vi "GV_Joystick1.vi"(8 "error in (no error)":errorcluster, 10 "device index":i32, 11 "Mode":enum16{"Init", "Destroy", "Read", "Change ID"}(ring)) -> (0 "error out":errorcluster, 1 "Connected?":bool, 2 "device":refnum<k1>, 3 "device ID":i32)   [LabVIEW 2012]
uses:
  <vilib>/Utility/inputDevices.llb/closeJoystick.vi
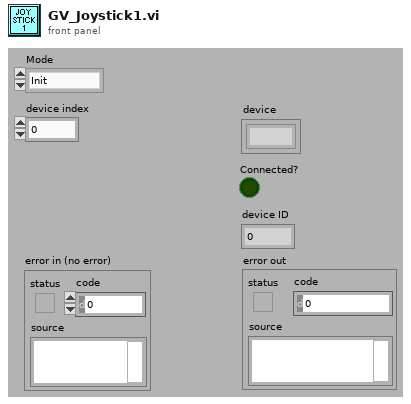
[diagram p1: front panel]
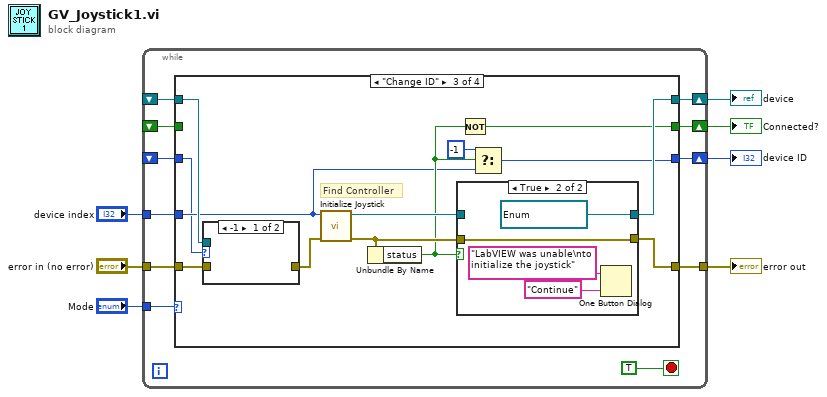
[diagram p0: block diagram]
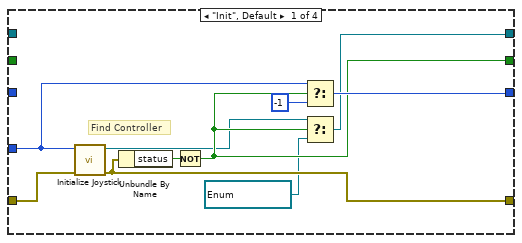
[diagram p2: hidden frame]
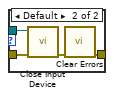
[diagram p4: hidden frame]
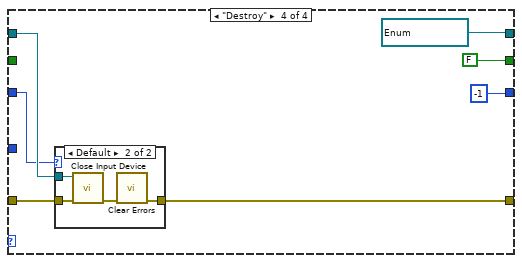
[diagram p6: hidden frame]
diagram:
  n1 = while {
    shift-right: [w18] -> w4
    shift-left: _ -> [w16]
    shift-right: [w17] -> w3
    shift-left: _ -> [w15]
    shift-right: [w13] -> w2
    shift-left: _ -> [w12]
    tunnel: "device index" -> [w11]
    tunnel: "Mode" -> [w10]
    tunnel: "error in (no error)" -> [w9]
    tunnel: [w8] -> w1
    stop <- TRUE stop-if-true
    n2 = case shown="\"Change ID\"" w10 {
      tunnel: [w20 w32 w43 w60] -> w18
      tunnel: [w22 w31 w41 FALSE] -> w17
      tunnel: w16 -> [_ w32 w40 w62]
      tunnel: w15 -> [_ w31 _ _]
      tunnel: w11 -> [w25 _ w34 _]
      tunnel: w9 -> [w27 w30 w39 w61]
      tunnel: [w28 w30 w42 w58] -> w8
      tunnel: [w23 w29 w36 -1 ("f")] -> w13
      tunnel: w12 -> [_ w29 w33 w56]
      frame "Init", Default {
        w19 = refnum<k1> refnum items=["JOYSTICK"] ("device ID")
        # "Find Controller"
        n3 = call <vilib>:"Initialize Joystick.vi"("error in (no error)"=w27, "device index"=w25) -> ("error out"=w28:errorcluster, "device ID"=w21:refnum<k1>)  [unwired: 8 in]
        n4 = Unbundle By Name(w28) -> ("status"=w26:bool)
        n5 = Not(x=w26) -> (.not. x?=w22:bool)
        n6 = Select(t=w25, s=w22, f=-1) -> (s? t:f=w23:i32)
        n7 = Select(t=w21, s=w22, f=w19) -> (s? t:f=w20:refnum<k1>)
      }
      frame "Read" {
      }
      frame "Change ID" {
        # "Find Controller"
        n8 = case shown="-1" w33 {
          tunnel: w40 -> [_ w49]
          tunnel: w39 -> [_ w48]
          tunnel: [_ w46] -> w38
          frame -1 {
          }
          frame Default {
            n9 = call-poly <vilib>:"Close Input Device.vi"("error in (no error)"=w48, "device ID"=w49) -> ("error out"=w47:errorcluster)  [unwired: 8 in]
            n10 = call <vilib>:"Clear Errors.vi"("error in (no error)"=w47) -> ("error out"=w46:errorcluster)  [unwired: 6 in]
          }
        }
        n11 = call <vilib>:"Initialize Joystick.vi"("error in (no error)"=w38, "device index"=w34) -> ("error out"=w45:errorcluster, "device ID"=w44:refnum<k1>)  [unwired: 8 in]
        n12 = Unbundle By Name(w45) -> ("status"=w37:bool)
        n13 = case shown="True" w37 {
          tunnel: w45 -> [w51 w53]
          tunnel: [w51 w53] -> w42
          tunnel: w44 -> [w50 _]
          tunnel: [w50 w52] -> w43
          frame False {
          }
          frame True {
            w52 = refnum<k1> refnum items=["JOYSTICK"] ("device ID")
            n14 = One Button Dialog(message="LabVIEW was unable\nto initialize the joystick", button name ("OK")="Continue") -> ()  [unwired: 1 out]
          }
        }
        n15 = Not(x=w37) -> (.not. x?=w41:bool)
        n16 = Select(t=-1 ("f"), s=w37, f=w34) -> (s? t:f=w36:i32)
      }
      frame "Destroy" {
        w60 = refnum<k1> refnum items=["JOYSTICK"] ("device ID")
        n17 = case shown="Default" w56 {
          tunnel: w62 -> [_ w67]
          tunnel: w61 -> [w63 w66]
          tunnel: [w63 w64] -> w58
          frame -1 {
          }
          frame Default {
            n18 = call-poly <vilib>:"Close Input Device.vi"("error in (no error)"=w66, "device ID"=w67) -> ("error out"=w65:errorcluster)  [unwired: 8 in]
            n19 = call <vilib>:"Clear Errors.vi"("error in (no error)"=w65) -> ("error out"=w64:errorcluster)  [unwired: 6 in]
          }
        }
      }
    }
  }
  "device" <- w4
  "Connected?" <- w3
  "device ID" <- w2
  "error out" <- w1
